vi "ModifiedRabiFlop1762WithPumpingHWT2cHIP.vi"() -> ()   [LabVIEW 2012]
uses:
  <vilib>/Utility/file.llb/Write To Spreadsheet File (DBL).vi
panel:
  out "Path 2":path=path "c:/data/1762 Scans/2014-05-20_19-16-05_1762scanWithPumping.txt"
  in  "Scrub the run?":bool=TRUE
  out "binned path":path=path "c:/data/1762 Scans/2015-04-16-Flops/2015-04-16_18-54-25_1762RabiPumped.txt"
  in  "Cooling Delay?":bool
  in  "Cooling Delay(ms)":u32
  in  "Heat Time(units of 1 us)":dbl
  in  "End (us)":dbl=50.0
  in  "Step (us)":dbl=10.0
  out "Current Time (us)":dbl=10.0
  in  "Start (us)":dbl
  in  "Frequency (MHz)":dbl=85.85
  out "digital waveform out 3":digitalwaveform(waveform)={"t0"=timestamp(0 s since 1904-01-01), "dt"=1e-07, "Y"={"transitions"=[0, 2100, 2200, 2300, 2301, 2411], "data"=[[1, 1, 1, 0, 0], [1, 0, 1, 0, 0], [1, 0, 0, 0, 0], [0, 0, 0, 0, 0], [0, 0, 0, 0, 0], [0, 1, 1, 0, 0]]}, "error"={"status"=FALSE, "code"=37421928, "source"=""}}
  out "10xwindow":i32
  out "10xdiscr":dbl
  out "DARK?":i32(graph)=50
  out "Counts":i32=50
  out "DARK?":bool
  out "PMT Counts":i32(graph)=42
  in  "PMT sample time":dbl=0.05
  out "Counts after 1762":i32=42
  out "OuterLoop":i32
  out "InnerLoop":i32=9
  out "Bright Events":dbl
  in  "Discriminator Level\n (Bright/Dark)":i32=70
  out "digital waveform out 2":digitalwaveform(waveform)={"t0"=timestamp(0 s since 1904-01-01), "dt"=1e-07, "Y"={"transitions"=[0, 2100, 2200, 2300, 2301, 2311, 2321, 2421], "data"=[[1, 1, 1, 0, 0], [1, 0, 1, 0, 0], [1, 0, 0, 0, 0], [0, 0, 0, 0, 0], [0, 0, 0, 0, 0], [0, 0, 0, 0, 1], [0, 0, 0, 0, 0], [0, 1, 1, 0, 0]]}, "error"={"status"=FALSE, "code"=37421928, "source"=""}}
  in  "Comment":string
  in  "B Field":dbl=2.91
  in  "RF Power":dbl=999.0
  out "Counts finding bright ion":dbl=50.0
  in  "BG Cutoff Limit":dbl=45.0
  in  "Runs per data point":dbl=50.0
  out "Path":path=path "c:/data/1762 Scans/2015-04-16_18-54-25_1762RabiPumped.txt"
  out "Frequency Scan":cluster{dbl, dbl}[](graph)=[{0.0, 0.8}]
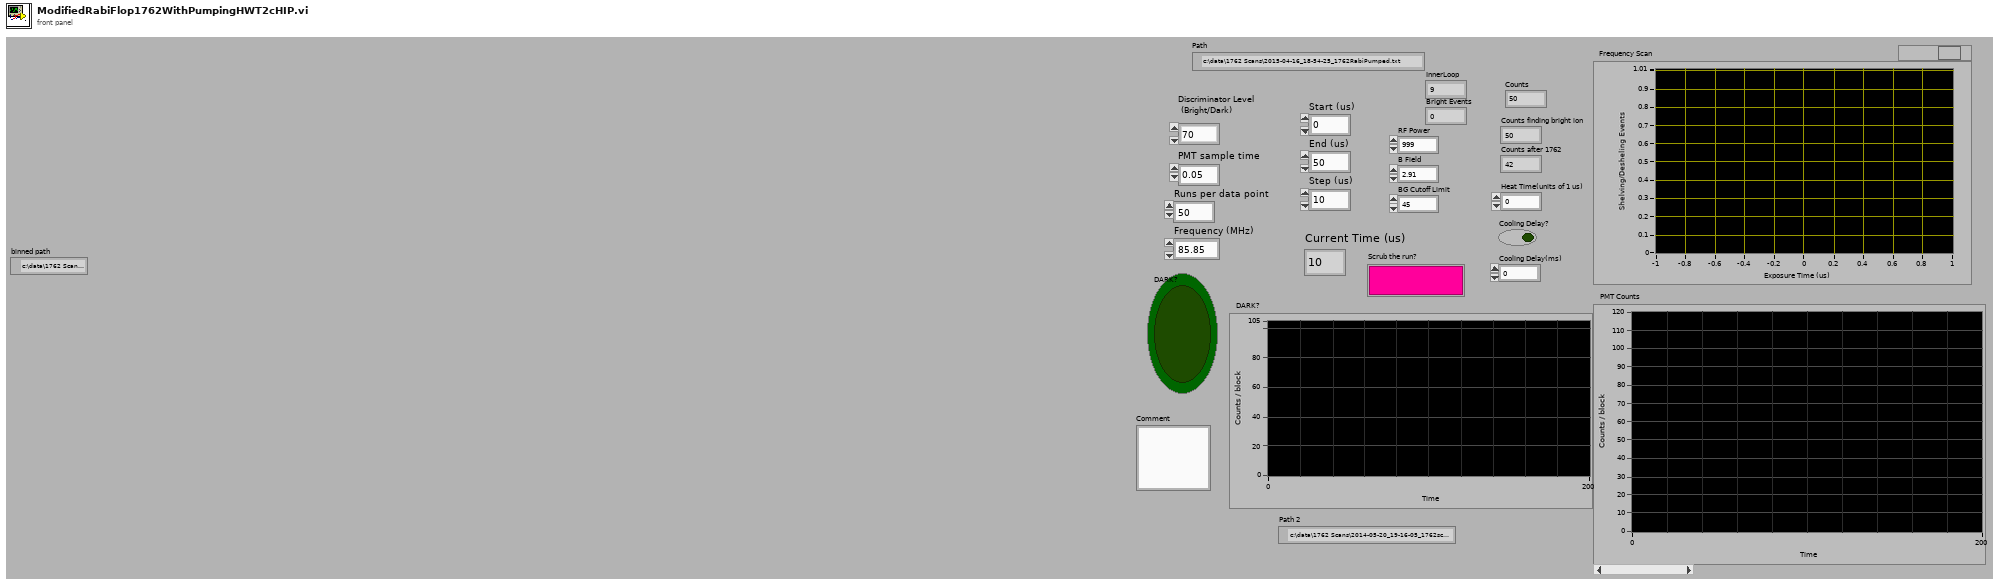
[diagram p1: front panel]
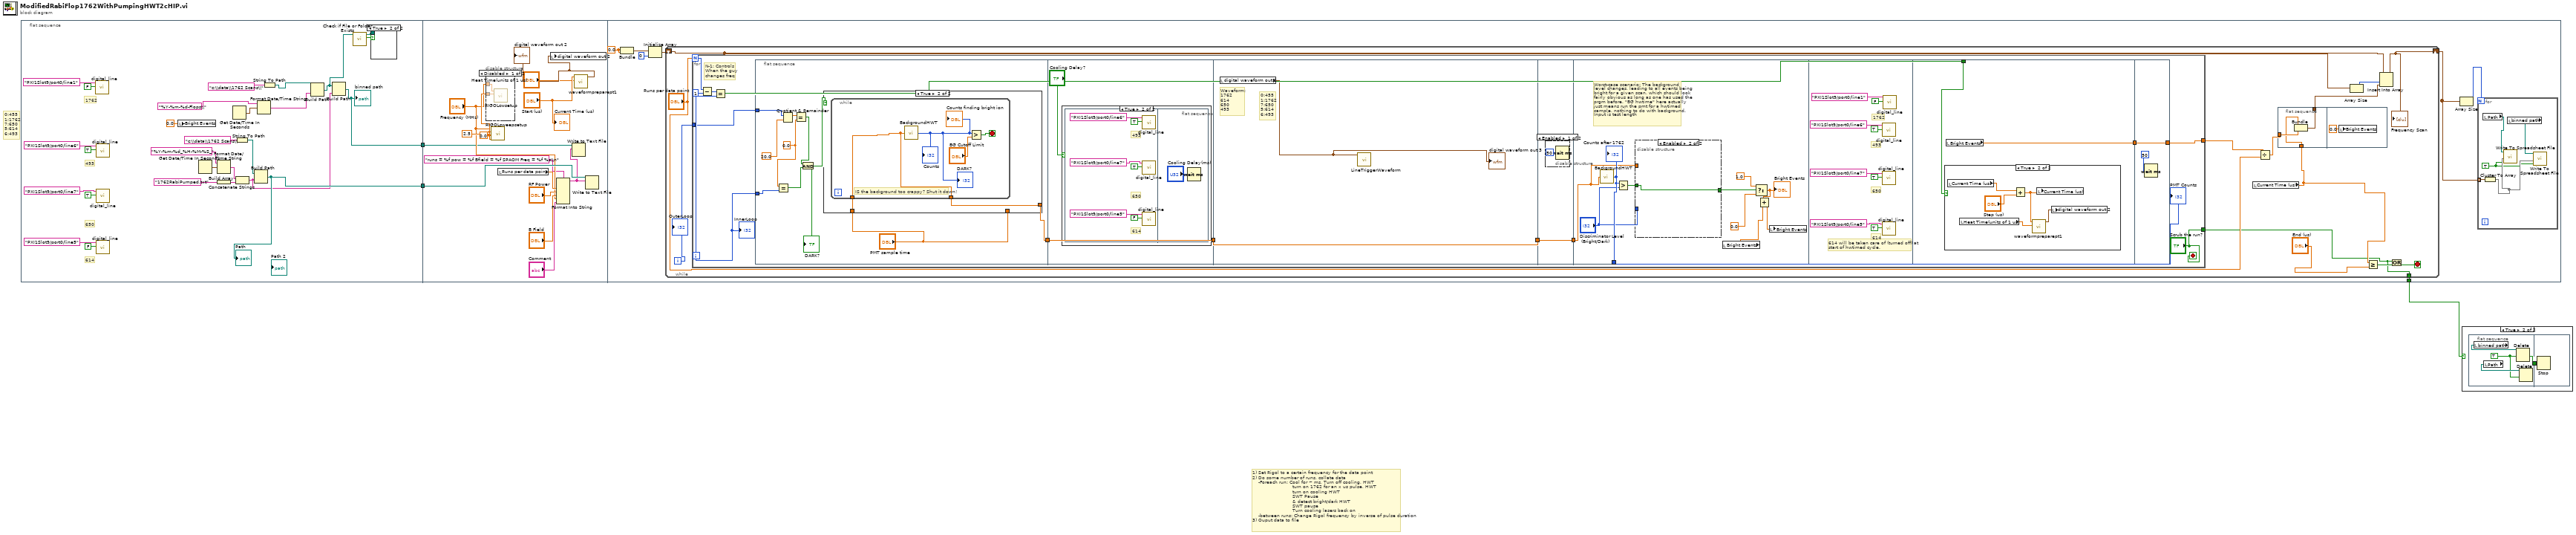
[diagram p0: block diagram]
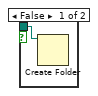
[diagram p3: hidden frame]
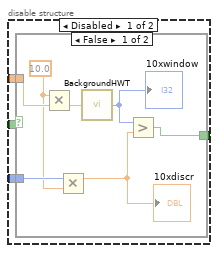
[diagram p8: hidden frame]
diagram:
  # "0:455\n1:1762\n7:650\n5:614\n6:493"
  # "1) Set Rigol to a certain frequency for the data point\n2) Do some number of runs, collate data\n    -Foreach run: Cool for ~ ms, Turn off cooling, HWT\n                           turn on 1762 for an x us pulse, HWT\n                           turn on cooling HWT\n                           SWT Pause\n                           & detect bright/dark HWT\n                           SWT pause\n                           Turn cooling lasers back on \n    -between runs: Change Rigol frequency by inverse of pulse duration\n3) Ouput data to file"
  n1 = flat-sequence {
    tunnel: [w23] -> w3
    tunnel: [w4] -> w2
    tunnel: w3 -> [w45]
    tunnel: w2 -> [w33]
    tunnel: [w48] -> w1
    frame #0 {
      # "614"
      # "650"
      # "493"
      # "1762"
      n2 = call "digital_line.vi"("Boolean"=FALSE, "lines"=tag "PXI1Slot9/port0/line1") -> ()  [unwired: 5 in, 1 out]
      n3 = call "digital_line.vi"("Boolean"=TRUE, "lines"=tag "PXI1Slot9/port0/line6") -> ()  [unwired: 5 in, 1 out]
      n4 = call "digital_line.vi"("Boolean"=TRUE, "lines"=tag "PXI1Slot9/port0/line7") -> ()  [unwired: 5 in, 1 out]
      n5 = call "digital_line.vi"("Boolean"=FALSE, "lines"=tag "PXI1Slot9/port0/line5") -> ()  [unwired: 5 in, 1 out]
      n6 = local write "Bright Events"(0.0 ("Bright Events")) -> ()
      n7 = Get Date/Time In Seconds() -> (seconds since 1Jan1904=w25:timestamp)
      n8 = Format Date/Time String(time format string (%c)="%Y-%m-%d_%H-%M-%S_", seconds (now)=w25) -> (date/time string=w27:string)  [unwired: 1 in]
      n9 = Build Array("1762RabiPumped.txt") -> (w29:string[])
      n10 = Get Date/Time In Seconds() -> (seconds since 1Jan1904=w12:timestamp)
      n11 = String To Path(string="c:\\data\\1762 Scans\\") -> (path=w30:path)
      n12 = Concatenate Strings(w27, w29) -> (w6:string)
      n13 = Build Path(base path=w30, name or relative path=w6) -> (appended path=w23:path)
      "Path" <- w23
      n14 = Format Date/Time String(time format string (%c)="%Y-%m-%d-Flops\\", seconds (now)=w12) -> (date/time string=w11:string)  [unwired: 1 in]
      n15 = String To Path(string="c:\\data\\1762 Scans\\") -> (path=w10:path)
      n16 = Build Path(base path=w10, name or relative path=w11) -> (appended path=w5:path)
      n17 = Build Path(base path=w5, name or relative path=w6) -> (appended path=w4:path)
      "binned path" <- w4
      n18 = call <vilib>:"Check if File or Folder Exists.vi"("path"=w5) -> ("file or folder exists?"=w9:bool, "dup path"=w8:path)  [unwired: 8 in, 1 out]
      n19 = case shown="True" w9 {
        tunnel: w8 -> [w31 _]
        frame False {
          n20 = Create Folder(path (use dialog)=w31) -> ()  [unwired: 2 in, 3 out]
        }
        frame True {
        }
      }
    }
    frame #1 {
      w38 = 0.0 ("Time (ms)")
      w39 = 2.5 ("Amplitude (Vpp)")
      n21 = disable-structure shown="Disabled" {
        disable-tunnel: w39 -> [w47 _]
        disable-tunnel: "Frequency (MHz)" -> [w46 _]
        frame Disabled {
          n22 = call "RIGOLcwsetup.vi"("Amplitude (Vpp)"=w47, "Frequency (MHz)"=w46) -> ()  [unwired: 10 in]
        }
        frame Enabled {
        }
      }
      n23 = call "RIGOLsweepsetup.vi"("AP Sweep Width (MHz)"=w38, "Time (ms)"=w38, "Amplitude (Vpp)"=w39, "Frequency (MHz)"="Frequency (MHz)") -> ()  [unwired: 8 in]
      n24 = local read "Runs per data point"() -> (w44:dbl)
      n25 = Format Into String(format string="runs = %f pow = %f Bfield = %f SPAOM Freq = %f %s\\n", w44, "RF Power", "B Field", "Frequency (MHz)", "Comment") -> (resulting string=w32:string)  [unwired: 2 in, 1 out]
      n26 = Write to Text File(file (use dialog)=w33, text=w32) -> ()  [unwired: 2 in, 3 out]
      n27 = call "waveformpreparept1.vi"("Heat Time(units of 1 us)"="Heat Time(units of 1 us)", "1762 pulse length (units of 1 us)"="Start (us)") -> ("digital waveform out 2"=w41:digitalwaveform)  [unwired: 7 in]
      "digital waveform out 2" <- w41
      n28 = local write "digital waveform out 2"(w41) -> ()
      n29 = Write to Text File(file (use dialog)=w45, text=w32) -> ()  [unwired: 2 in, 3 out]
      "Current Time (us)" <- "Start (us)"
    }
    frame #2 {
      w53 = 0.0
      n30 = Bundle(w53, w53) -> (w54:cluster{dbl, dbl})  [unwired: 1 in]
      n31 = Initialize Array(w54, 0) -> (w51:cluster{dbl, dbl}[])
      n32 = while {
        shift-right: [w69] -> w49
        shift-left: w51 -> [w70]
        tunnel: [w60] -> w48
        i -> [w68]
        stop <- w61 stop-if-true
        n33 = for {
          N: "Runs per data point" -> [w87]
          tunnel: [w86] -> w66
          tunnel: w68 -> [w83]
          tunnel: ["Scrub the run?"] -> w60
          i -> [w84]
          stop <- "Scrub the run?" stop-if-true
          # "N-1: Controls\nWhen the guy\nchanges freq"
          n34 = Subtract(x=w87, y=1) -> (x-y=w90:i32)
          n35 = Equal?(x=w90, y=w84) -> (x = y?=w88:bool)
          n36 = flat-sequence {
            tunnel: w84 -> [w98]
            tunnel: w83 -> [w93]
            tunnel: [w92] -> w79
            tunnel: w79 -> [w109]
            tunnel: [w109] -> w78
            tunnel: [w118] -> w80
            tunnel: w78 -> [w118]
            tunnel: [w119] -> w81
            tunnel: w80 -> [w119]
            tunnel: w81 -> [w123]
            tunnel: [w125] -> w82
            tunnel: w88 -> [w152]
            tunnel: [w153] -> w85
            tunnel: [w160] -> w86
            tunnel: w85 -> [w160]
            frame #0 {
              w97 = 0.0 ("x")
              n37 = Equal?(x=w97, y=w98) -> (x = y?=w95:bool)
              n38 = Quotient & Remainder(x=w93, y=20.0 ("Rerun BG Every\nnth freq point")) -> (x-y*floor(x/y)=w99:dbl)  [unwired: 1 out]
              n39 = Equal?(x=w99, y=w97) -> (x = y?=w96:bool)
              n40 = And(x=w96, y=w95) -> (x .and. y?=w94:bool)
              "DARK?" <- w94
              n41 = case shown="True" w94 {
                tunnel: [w101 w103] -> w92
                tunnel: "PMT sample time" -> [w101 _]
                tunnel: "PMT sample time" -> [_ w102]
                frame False {
                }
                frame True {
                  n42 = while {
                    tunnel: [w104] -> w103
                    tunnel: w102 -> [w104]
                    stop <- w106 stop-if-true
                    # "IS the background too crappy? Shut it down!"
                    n43 = call "BackgroundHWT.vi"("Sample Time(seconds)"=w104) -> ("Counts"=w105:i32)
                    "Counts finding bright ion" <- w105
                    "Counts" <- w105
                    "DARK?" <- w105
                    n44 = Greater?(x=w105, y="BG Cutoff Limit") -> (0:w106:bool)
                  }
                }
              }
            }
            frame #1 {
              n45 = case shown="True" "Cooling Delay?" {
                frame False {
                }
                frame True {
                  n46 = flat-sequence {
                    frame #0 {
                      # "614"
                      # "650"
                      # "493"
                      n47 = call "digital_line.vi"("Boolean"=TRUE, "lines"=tag "PXI1Slot9/port0/line6") -> ()  [unwired: 5 in, 1 out]
                      n48 = call "digital_line.vi"("Boolean"=TRUE, "lines"=tag "PXI1Slot9/port0/line7") -> ()  [unwired: 5 in, 1 out]
                      n49 = call "digital_line.vi"("Boolean"=FALSE, "lines"=tag "PXI1Slot9/port0/line5") -> ()  [unwired: 5 in, 1 out]
                    }
                    frame #1 {
                      n50 = Wait (ms)(milliseconds to wait="Cooling Delay(ms)") -> ()  [unwired: 1 out]
                    }
                  }
                }
              }
            }
            frame #2 {
              # "0:455\n1:1762\n7:650\n5:614\n6:493"
              # "Waveform:\n1762\n614\n650\n493"
              n51 = local read "digital waveform out 2"() -> (w117:digitalwaveform)
              "digital waveform out 3" <- w117
              n52 = call "LineTriggerWaveform.vi"("digital waveform in"=w117) -> ()  [unwired: 11 in]
            }
            frame #3 {
              n53 = disable-structure shown="Enabled" {
                frame Enabled {
                  n54 = Wait (ms)(milliseconds to wait=u32 50) -> ()  [unwired: 1 out]
                }
                frame Disabled {
                }
              }
            }
            frame #4 {
              # "Worst-case scenario: The background\nlevel changes, leading to all events being\nbright for a given scan, which should look\nfairly obvious as long as one has used the\nprgm before. \"BG hwtime\" here actually\njust means run the pmt for a hwtimed\nsample, nothing to do with background.\nInput is test length"
              n55 = call "BackgroundHWT.vi"("Sample Time(seconds)"=w123) -> ("Counts"=w125:i32)
              "Counts after 1762" <- w125
              n56 = Greater?(x=w125, y="Discriminator Level\n (Bright/Dark)") -> (0:w124:bool)
              n57 = disable-structure shown="Enabled" {
                disable-tunnel: w124 -> [w134 w143]
                disable-tunnel: [w133 w143] -> w121
                disable-tunnel: w123 -> [w132 _]
                disable-tunnel: "Discriminator Level\n (Bright/Dark)" -> [w131 _]
                frame Disabled {
                  n58 = case shown="False" w134 {
                    selector: w134 -> [_ w142]
                    tunnel: [w137 w142] -> w133
                    tunnel: w132 -> [w141 _]
                    tunnel: w131 -> [w138 _]
                    frame False {
                      w135 = 10.0 ("x")
                      n59 = Multiply(x=w135, y=w141) -> (x*y=w140:dbl)
                      n60 = Multiply(x=w138, y=w135) -> (x*y=w136:dbl)
                      "10xdiscr" <- w136
                      n61 = call "BackgroundHWT.vi"("Sample Time(seconds)"=w140) -> ("Counts"=w139:i32)
                      "10xwindow" <- w139
                      n62 = Greater?(x=w139, y=w136) -> (0:w137:bool)
                    }
                    frame True {
                    }
                  }
                }
                frame Enabled {
                }
              }
              n63 = local read "Bright Events"() -> (w126:dbl)
              n64 = Select(t=1.0, s=w121, f=0.0) -> (s? t:f=w128:dbl)
              "Bright Events" <- w128
              n65 = Add(x=w128, y=w126) -> (x+y=w127:dbl)
              n66 = local write "Bright Events"(w127) -> ()
            }
            frame #5 {
              # "614 will be taken care of (turned off) at\nstart of hwtimed cycle."
              # "614"
              # "650"
              # "493"
              # "1762"
              n67 = call "digital_line.vi"("Boolean"=TRUE, "lines"=tag "PXI1Slot9/port0/line6") -> ()  [unwired: 5 in, 1 out]
              n68 = call "digital_line.vi"("Boolean"=TRUE, "lines"=tag "PXI1Slot9/port0/line7") -> ()  [unwired: 5 in, 1 out]
              n69 = call "digital_line.vi"("Boolean"=TRUE, "lines"=tag "PXI1Slot9/port0/line5") -> ()  [unwired: 5 in, 1 out]
              n70 = call "digital_line.vi"("Boolean"=FALSE, "lines"=tag "PXI1Slot9/port0/line1") -> ()  [unwired: 5 in, 1 out]
            }
            frame #6 {
              n71 = case shown="True" w152 {
                frame False {
                }
                frame True {
                  n72 = local read "Current Time (us)"() -> (w158:dbl)
                  n73 = local read "Heat Time(units of 1 us)"() -> (w154:dbl)
                  n74 = Add(x=w158, y="Step (us)") -> (x+y=w156:dbl)
                  n75 = call "waveformpreparept1.vi"("Heat Time(units of 1 us)"=w154, "1762 pulse length (units of 1 us)"=w156) -> ("digital waveform out 2"=w155:digitalwaveform)  [unwired: 7 in]
                  n76 = local write "Current Time (us)"(w156) -> ()
                  n77 = local write "digital waveform out 2"(w155) -> ()
                }
              }
              n78 = local read "Bright Events"() -> (w153:dbl)
            }
            frame #7 {
              n79 = Wait (ms)(milliseconds to wait=u32 50) -> ()  [unwired: 1 out]
            }
          }
          "InnerLoop" <- w84
          "PMT Counts" <- w82
        }
        n80 = local read "Current Time (us)"() -> (w63:dbl)
        n81 = Divide(x=w66, y="Runs per data point") -> (x/y=w65:dbl)
        n82 = flat-sequence {
          tunnel: w65 -> [w75]
          tunnel: [w74] -> w67
          tunnel: w63 -> [w73]
          frame #0 {
            n83 = Bundle("Current Time (us)"=w73, w75) -> (w74:cluster{"Current Time (us)":dbl, dbl})  [unwired: 1 in]
          }
          frame #1 {
            n84 = local write "Bright Events"(0.0 ("Bright Events")) -> ()
          }
        }
        n85 = Array Size(array=w70) -> (size(s)=w71:i32)
        n86 = Greater Or Equal?(x=w63, y="End (us)") -> (x >= y?=w72:bool)
        n87 = Insert Into Array(array=w70, index=w71, new element=w67) -> (w69:cluster{dbl, dbl}[])
        "Frequency Scan" <- w69
        n88 = Or(x=w60, y=w72) -> (x .or. y?=w61:bool)
        "OuterLoop" <- w68
      }
      n89 = Array Size(array=w49) -> (size(s)=w50:i32)
      n90 = for {
        N: w50 -> [_]
        tunnel: w49 -> [w59] mode=indexing
        w55 = TRUE
        n91 = local read "Path"() -> (w58:path)
        n92 = Cluster To Array(cluster=w59) -> (array=w56:dbl[])
        n93 = call-poly <vilib>:"Write To Spreadsheet File.vi"("append to file? (new file:F)"=w55, "1D data"=w56, "file path (dialog if empty)"=w58) -> ()  [unwired: 5 in, 1 out]
        n94 = local read "binned path"() -> (w57:path)
        n95 = call-poly <vilib>:"Write To Spreadsheet File.vi"("append to file? (new file:F)"=w55, "1D data"=w56, "file path (dialog if empty)"=w57) -> ()  [unwired: 5 in, 1 out]
      }
    }
  }
  n96 = case shown="True" w1 {
    frame False {
    }
    frame True {
      n97 = flat-sequence {
        tunnel: [w163] -> w161
        tunnel: w161 -> [w166]
        frame #0 {
          w162 = TRUE
          n98 = local read "binned path"() -> (w165:path)
          n99 = local read "Path"() -> (w164:path)
          n100 = Delete(path (use dialog)=w165, confirm (F)=w162) -> (cancelled=w163:bool)  [unwired: 3 in, 2 out]
          n101 = Delete(path (use dialog)=w164, confirm (F)=w162) -> ()  [unwired: 3 in, 3 out]
        }
        frame #1 {
          n102 = Stop(stop? (T)=w166) -> ()
        }
      }
    }
  }
